vi "Velocity Correction.vi"(0 "raw impact":sgl format="%.3f", 1 "distance units":string="SI", 5 "raw redundant":sgl format="%.3f", 7 "raw residual":sgl=1.0 format="%.3f", 9 "screen set midpt to target":sgl format="%.3f", 11 "residual screen to target":sgl format="%.3f", 12 "correction coefficient":sgl format="%.5f") -> (4 "corrected impact":sgl format="%.3f", 6 "corrected redundant":sgl format="%.3f", 8 "corrected residual":sgl=1.0 format="%.3f", 10 "impact factor":sgl=1.0 format="%.4f", 14 "conversion factor":sgl format="%.5f", 15 "residual factor":sgl format="%.4f")   [LabVIEW 2015]
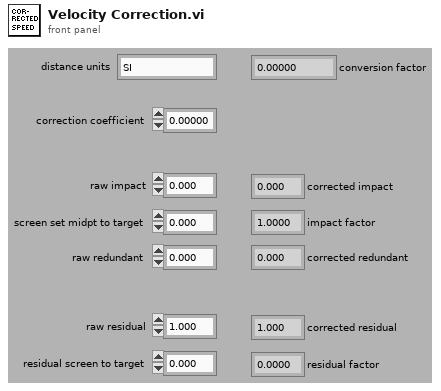
[diagram p1: front panel]
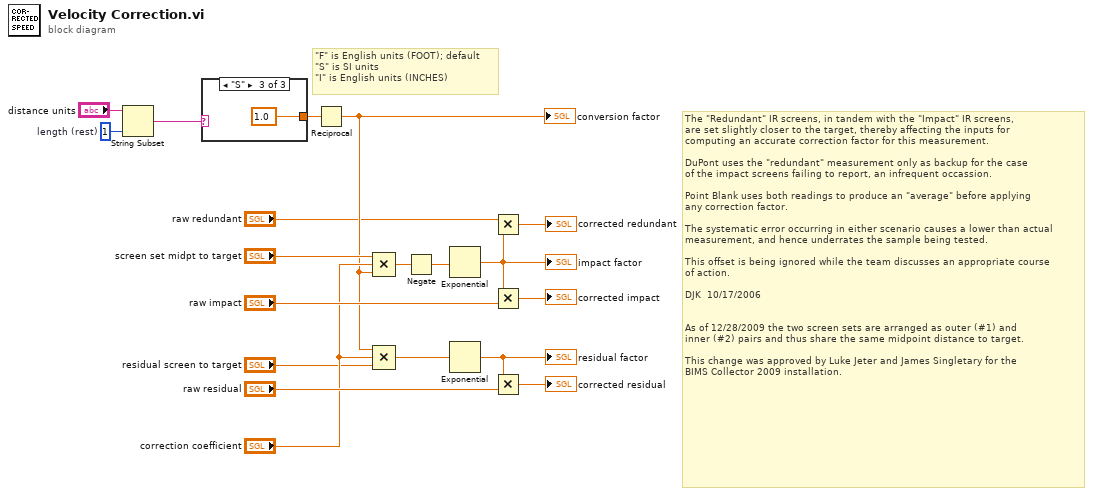
[diagram p0: block diagram]
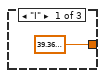
[diagram p2: hidden frame]
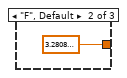
[diagram p3: hidden frame]
diagram:
  w18 = 1  # length (rest)
  # "\"F\" is English units (FOOT); default\n\"S\" is SI units\n\"I\" is English units (INCHES)"
  # "The \"Redundant\" IR screens, in tandem with the \"Impact\" IR screens,\nare set slightly closer to the target, thereby affecting the inputs for \ncomputing an accurate correction factor for this measurement.\n\nDuPont uses the \"redundant\" measurement only as backup for the case \nof the impact screens failing to report, an infrequent occassion.\n\nPoint Blank uses both readings to produce an \"average\" before applying \nany correction factor.\n\nThe systematic error occurring in either scenario causes a lower than actual \nmeasurement, and hence underrates the sample being tested.\n\nThis offset is being ignored while the team discusses an appropriate course \nof action.\n\nDJK  10/17/2006\n\n\nAs of 12/28/2009 the two screen sets are arranged as outer (#1) and \ninner (#2) pairs and thus share the same midpoint distance to target. \n\nThis change was approved by Luke Jeter and James Singletary for the \nBIMS Collector 2009 installation."
  n1 = String Subset(string="distance units", length (rest)=w18) -> (substring=w17:string)  [unwired: 1 out]
  n2 = case shown="\"S\"" w17 {
    tunnel: [sgl 39.37 sgl 3.2808 sgl 1.0] -> w8
    frame "I" {
    }
    frame "F", Default {
    }
    frame "S" {
    }
  }
  n3 = Reciprocal(x=w8) -> (1/x=w4:sgl)
  "conversion factor" <- w4
  n4 = Compound Arithmetic op=MULTIPLY("screen set midpt to target", "correction coefficient", w4) -> (w16:sgl)
  n5 = Compound Arithmetic op=MULTIPLY(w4, "correction coefficient", "residual screen to target") -> (w12:sgl)
  n6 = Negate(x=w16) -> (-x=w15:sgl)
  n7 = Exponential(1:w15) -> (0:w3:sgl)
  "impact factor" <- w3
  n8 = Exponential(1:w12) -> (0:w11:sgl)
  "residual factor" <- w11
  n9 = Multiply(x="raw redundant", y=w3) -> (x*y=→"corrected redundant":sgl)
  n10 = Multiply(x=w3, y="raw impact") -> (x*y=→"corrected impact":sgl)
  n11 = Multiply(x=w11, y="raw residual") -> (x*y=→"corrected residual":sgl)
